vi "Tiles2004.vi"   [LabVIEW 2013]
uses:
  <vilib>/Heliosphere Research LLC/Advanced Plotting Toolkit/Advanced Plotting Toolkit.lvlib
types:
  T1 = typedef "Advanced Plotting Toolkit.lvlib/PlotID.ctl" = i32
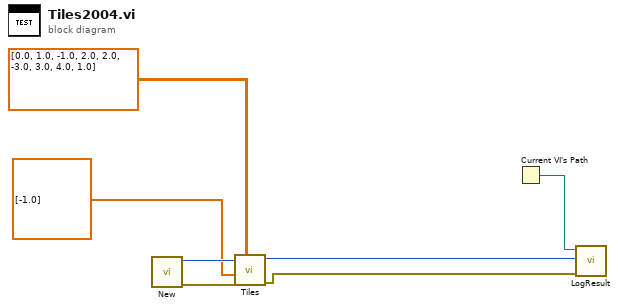
[diagram p0: block diagram]
diagram:
  n1 = call <vilib>:"New.vi"() -> ("error out"=w5:errorcluster, "Plot ID"=w4:T1)  [unwired: 10 in]
  n2 = call <vilib>:"Tiles.vi"("Z Data"=dbl[][] [[0.0, 1.0, -1.0], [2.0, 2.0, -3.0], [3.0, 4.0, 1.0]], "error in (no error)"=w5, "Y Tile Boundaries"=dbl[] [-1.0] ("X Tile Boundaries"), "Plot ID"=w4) -> ("error out"=w3:errorcluster, "Plot ID Out"=w2:T1)  [unwired: 6 in]
  n3 = Current VI's Path() -> (path=w7:path)
  n4 = call "LogResult.vi"("Test Result"=w3, "Test Artifact"=w2, "VI Path"=w7) -> ()  [unwired: 9 in]
